vi "Initialize Device.vi"(7 "Baud Rate Override":u32, 8 "Error In":errorcluster, 9 "TCP Configuration":T3, 10 "COM Port":refnum<visa-resource-name>, 11 "Interface":T2) -> (0 "Error Out":errorcluster, 3 "LINX Device Config":T1)   [LabVIEW 2020, in "Device.lvlib"]
doc: "Open a connection to the LINX device."
uses:
  Device.lvlib
  Type Defs/TCP Config.ctl
  Type Defs/Interface.ctl
  Type Defs/LINX Device Config.ctl
  Type Defs/Channels.ctl
  Type Defs/Packet Number FGV Action.ctl
  LMH-LINX.lvlib
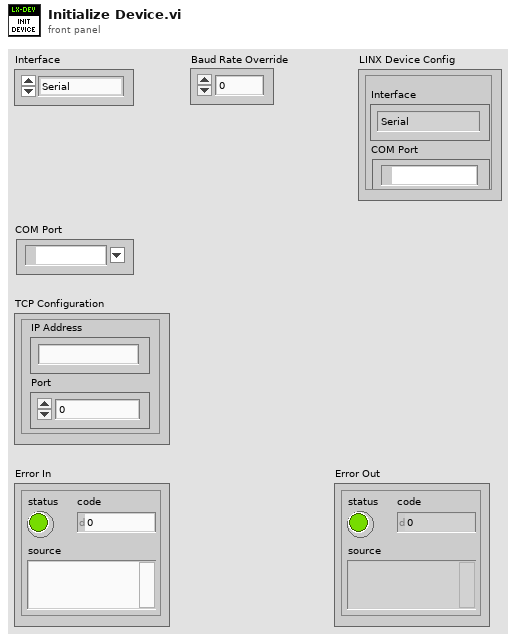
[diagram p1: front panel]
types:
  T1 = typedef "Device.lvlib/LINX Device Config.ctl" = cluster{"Interface":T2, "COM Port":refnum<visa-resource-name>, "TCP Configuration":T3, "Device Family":u8, "Device ID":u8, "Device Name":string, "TCP Ref":refnum<k5>, "Channels":T4}
  T2 = typedef "LMH-LINX.lvlib/Interface.ctl" = enum16{"Serial", "TCP"}
  T3 = typedef "Device.lvlib/TCP Config.ctl" = cluster{"IP Address":string, "Port":u16}
  T4 = typedef "LMH-LINX.lvlib/Channels.ctl" = cluster{"DI":u8[], "DO":u8[], "AI":u8[], "AO":u8[], "PWM":u8[], "QE":u8[], "UART":u8[], "I2C 2":u8[], "SPI":u8[], "CAN":u8[], "Servo":u8[], "AI Ref (V)":dbl, "AI Resolution (Bits)":u8, "AO Ref (V)":dbl, "AO Resolution (Bits)":u8}
  T5 = typedef "Device.lvlib/Packet Number FGV Action.ctl" = enum16{"Initialize", "Get", "Increment"}
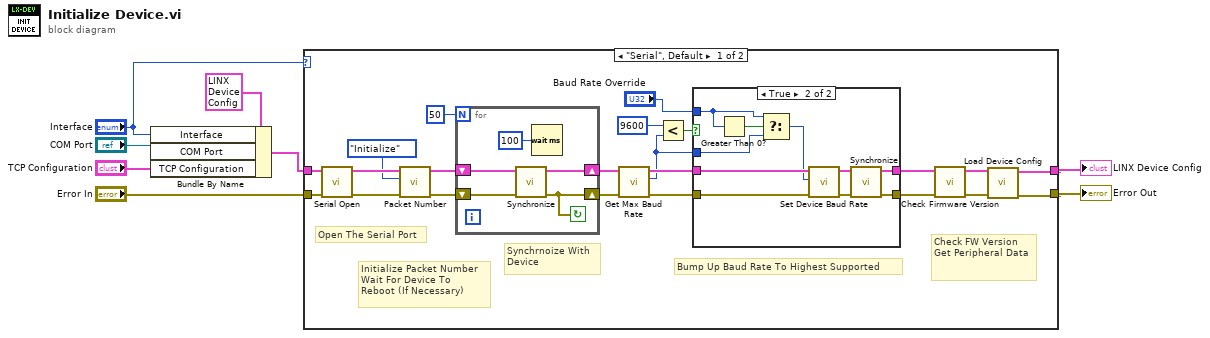
[diagram p0: block diagram]
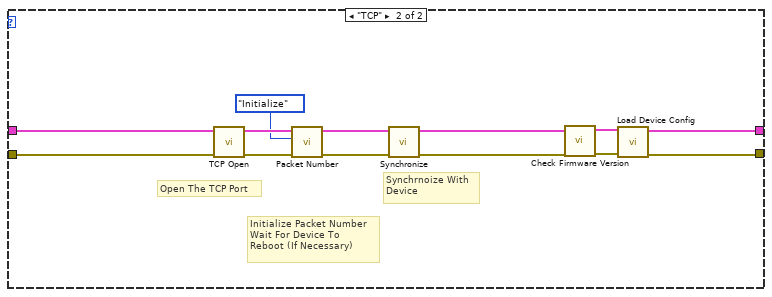
[diagram p3: hidden frame]
diagram:
  n1 = Bundle By Name(cluster=T1 {"Interface"=enum."Serial", "COM Port"="", "TCP Configuration"={"IP Address"="", "Port"=0}, "Device Family"=0, "Device ID"=0, "Device Name"="", "TCP Ref"=refnum, "Channels"={"DI"=[], "DO"=[], "AI"=[], "AO"=[], "PWM"=[], "QE"=[], "UART"=[], "I2C 2"=[], "SPI"=[], "CAN"=[], "Servo"=[], "AI Ref (V)"=0.0, "AI Resolution (Bits)"=0, "AO Ref (V)"=0.0, "AO Resolution (Bits)"=0}} ("LINX Device Config"), "Interface"="Interface", "COM Port"="COM Port", "TCP Configuration"="TCP Configuration") -> (w3:T1)
  n2 = case shown="\"Serial\", Default" "Interface" {
    tunnel: "Error In" -> [w30 w60]
    tunnel: [w23 w53] -> w1
    tunnel: w3 -> [w29 w59]
    tunnel: [w24 w54] -> w2
    frame "Serial", Default {
      # "Initialize Packet Number\nWait For Device To \nReboot (If Necessary)"
      # "Check FW Version\nGet Peripheral Data"
      # "Bump Up Baud Rate To Highest Supported"
      # "Synchrnoize With\nDevice"
      # "Open The Serial Port"
      n3 = call "Serial Open.vi"("Error In"=w30, "LINX Device Config"=w29) -> ("Error Out"=w25:errorcluster, "LINX Device Config"=w28:T1)  [unwired: 8 in]
      n4 = call "Packet Number.vi"("Error In"=w25, "Action"=Packet_Number_FGV_Action."Initialize", "LINX Device Config"=w28) -> ("Error Out"=w26:errorcluster, "LINX Device Config"=w27:T1)  [unwired: 6 in, 1 out]
      n5 = for {
        N: 50 -> [_]
        shift-right: [w33] -> w22
        shift-left: w27 -> [w35]
        shift-right: [w32] -> w21
        shift-left: w26 -> [w34]
        stop <- w32 continue-if-true
        n6 = call "Synchronize.vi"("Error In"=w34, "LINX Device Config"=w35) -> ("Error Out"=w32:errorcluster, "LINX Device Config"=w33:T1)  [unwired: 8 in]
        n7 = Wait (ms)(milliseconds to wait=u32 100) -> ()  [unwired: 1 out]
      }
      n8 = call "Get Max Baud Rate.vi"("Error In"=w21, "LINX Device Config"=w22) -> ("Error Out"=w17:errorcluster, "Baud Rate"=w14:u32, "LINX Device Config"=w18:T1)  [unwired: 7 in]
      n9 = Less?(x=u32 9600 ("y"), y=w14) -> (x < y?=w15:bool)
      n10 = case shown="True" w15 {
        tunnel: w18 -> [w37 w47]
        tunnel: w17 -> [w36 w46]
        tunnel: [w37 w43] -> w20
        tunnel: [w36 w42] -> w19
        tunnel: w14 -> [_ w40]
        tunnel: "Baud Rate Override" -> [_ w38]
        frame False {
          # "No Faster Baud Rates Supported"
        }
        frame True {
          n11 = Greater Than 0?(x=w38) -> (x > 0?=w41:bool)
          n12 = Select(t=w38, s=w41, f=w40) -> (s? t:f=w39:u32)
          n13 = call "Set Device Baud Rate.vi"("Error In"=w46, "Baud Rate"=w39, "LINX Device Config"=w47) -> ("Error Out"=w44:errorcluster, "LINX Device Config"=w45:T1)  [unwired: 6 in, 1 out]
          n14 = call "Synchronize.vi"("Error In"=w44, "LINX Device Config"=w45) -> ("Error Out"=w42:errorcluster, "LINX Device Config"=w43:T1)  [unwired: 8 in]
        }
      }
      n15 = call "Check Firmware Version.vi"("Error In"=w19, "LINX Device Config"=w20) -> ("Error Out"=w13:errorcluster, "LINX Device Config"=w12:T1)  [unwired: 8 in]
      n16 = call "Load Device Config.vi"("Error In"=w13, "LINX Device Config"=w12) -> ("Error Out"=w23:errorcluster, "LINX Device Config"=w24:T1)  [unwired: 8 in]
    }
    frame "TCP" {
      # "Synchrnoize With\nDevice"
      # "Initialize Packet Number\nWait For Device To \nReboot (If Necessary)"
      # "Open The TCP Port"
      n17 = call "TCP Open.vi"("Error In"=w60, "LINX Device Config"=w59) -> ("Error Out"=w55:errorcluster, "LINX Device Config"=w58:T1)  [unwired: 8 in]
      n18 = call "Packet Number.vi"("Error In"=w55, "Action"=Packet_Number_FGV_Action."Initialize", "LINX Device Config"=w58) -> ("Error Out"=w56:errorcluster, "LINX Device Config"=w57:T1)  [unwired: 6 in, 1 out]
      n19 = call "Synchronize.vi"("Error In"=w56, "LINX Device Config"=w57) -> ("Error Out"=w48:errorcluster, "LINX Device Config"=w49:T1)  [unwired: 8 in]
      n20 = call "Check Firmware Version.vi"("Error In"=w48, "LINX Device Config"=w49) -> ("Error Out"=w51:errorcluster, "LINX Device Config"=w50:T1)  [unwired: 8 in]
      n21 = call "Load Device Config.vi"("Error In"=w51, "LINX Device Config"=w50) -> ("Error Out"=w53:errorcluster, "LINX Device Config"=w54:T1)  [unwired: 8 in]
    }
  }
  "Error Out" <- w1
  "LINX Device Config" <- w2
